vi "AlliGator Set Phasor Ratio Display Range.vi"(8 "error in (no error)":errorcluster, 11 "Phasor Ratio Display Range":refnum<vi>) -> (0 "error out":errorcluster)   [LabVIEW 2021, in "AlliGator Settings.lvlib"]
doc: "Constrains the sliders of the Phasor Ratio (or other parameter) Range to the displayed slide's min and max values."
uses:
  AlliGator Settings.lvlib
panel:
  # "see the AlliGator License on the block diagram (Ctrl+E or Window:Show Block Diagram)"
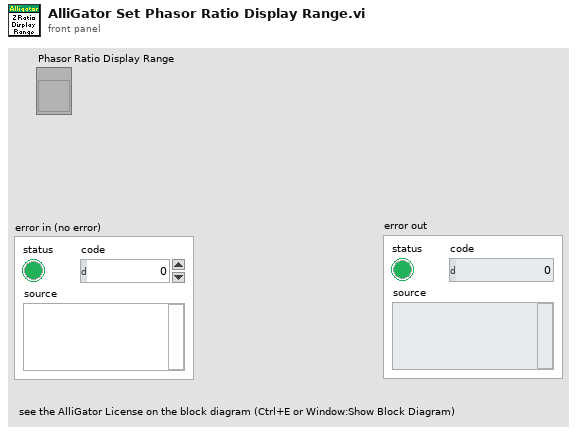
[diagram p1: front panel]
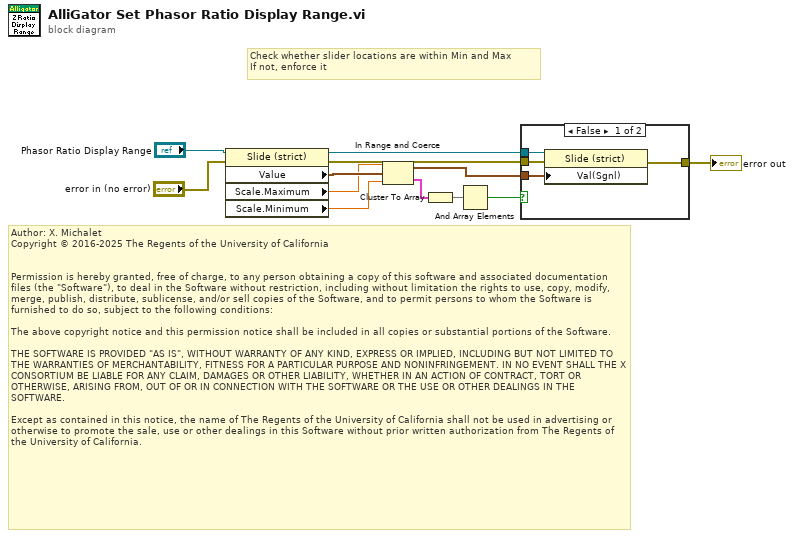
[diagram p0: block diagram]
diagram:
  # "Author: X. Michalet\nCopyright © 2016-2025 The Regents of the University of California\n \n\nPermission is hereby granted, free of charge, to any person obtaining a copy of this software and associated documentation files (the \"Software\"), to deal in the Software without restriction, including without limitation the rights to use, copy, modify, merge, publish, distribute, sublicense, and/or sell copies of the Software, and to permit persons to whom the Software is furnished to do so, subject to the following conditions:\n\nThe above copyright notice and this permission notice shall be included in all copies or substantial portions of the Software.\n\nTHE SOFTWARE IS PROVIDED \"AS IS\", WITHOUT WARRANTY OF ANY KIND, EXPRESS OR IMPLIED, INCLUDING BUT NOT LIMITED TO THE WARRANTIES OF MERCHANTABILITY, FITNESS FOR A PARTICULAR PURPOSE AND NONINFRINGEMENT. IN NO EVENT SHALL THE X CONSORTIUM BE LIABLE FOR ANY CLAIM, DAMAGES OR OTHER LIABILITY, WHETHER IN AN ACTION OF CONTRACT, TORT OR OTHERWISE, ARISING FROM, OUT OF OR IN CONNECTION WITH THE SOFTWARE OR THE USE OR OTHER DEALINGS IN THE SOFTWARE.\n\nExcept as contained in this notice, the name of The Regents of the University of California shall not be used in advertising or otherwise to promote the sale, use or other dealings in this Software without prior written authorization from The Regents of the University of California."
  # "Check whether slider locations are within Min and Max\nIf not, enforce it"
  n1 = property class="Slide (strict)"(reference="Phasor Ratio Display Range", error in="error in (no error)") -> (reference out=w3:refnum<vi>, error out=w2:errorcluster, "Value"=w10:cluster{dbl, dbl}, "Scale.Maximum"=w9:dbl, "Scale.Minimum"=w8:dbl)
  n2 = In Range and Coerce(upper limit=w9, x=w10, lower limit=w8) -> (coerced(x)=w7:cluster{dbl, dbl}, In Range?=w6:cluster{bool, bool})
  n3 = Cluster To Array(cluster=w6) -> (array=w5:bool[])
  n4 = And Array Elements(Boolean array=w5) -> (logical AND=w4:bool)
  n5 = case shown="False" w4 {
    tunnel: w7 -> [w16 _]
    tunnel: w3 -> [w15 _]
    tunnel: w2 -> [w14 w17]
    tunnel: [w13 w17] -> w1
    frame False {
      n6 = property class="Slide (strict)"(reference=w15, error in=w14, "Val(Sgnl)"=w16) -> (error out=w13:errorcluster)  [unwired: 1 out]
    }
    frame True {
    }
  }
  "error out" <- w1
